vi "MagState.vi"(8 "Error in":errorcluster, 11 "Serial port":refnum<visa-resource-name>="COM28") -> (0 "Error out":errorcluster, 2 "Mag State":bool[](array[boolean]), 3 "Serial port out":refnum<visa-resource-name>)   [LabVIEW 2012]
panel:
  out "State Value":i8[](array[numeric])
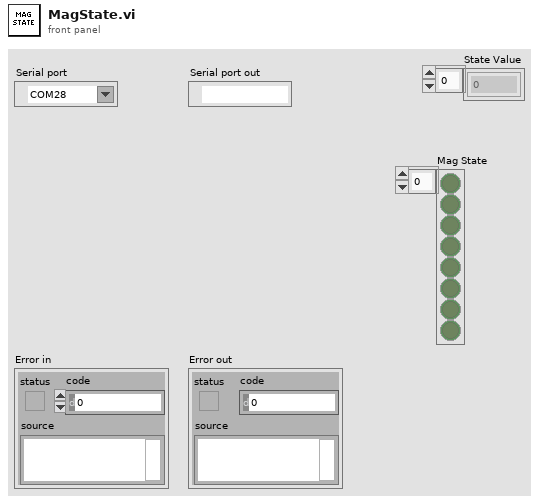
[diagram p1: front panel]
types:
  T1 = enum16{"big-endian, network order", "native, host order", "little-endian"}
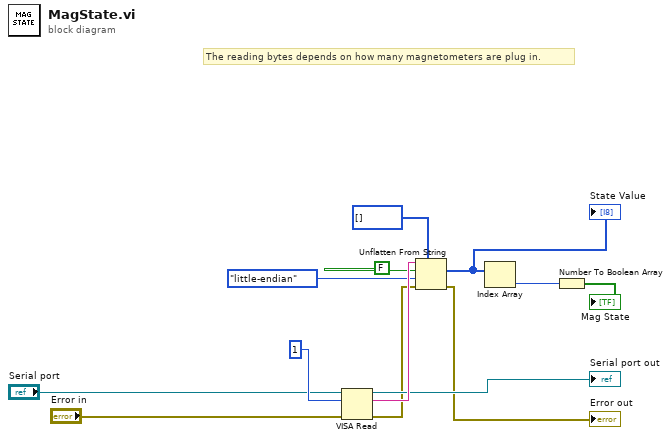
[diagram p0: block diagram]
diagram:
  # "The reading bytes depends on how many magnetometers are plug in."
  n1 = VISA Read(VISA resource name="Serial port", byte count=u32 1, error in (no error)="Error in") -> (VISA resource name out=→"Serial port out":refnum<visa-resource-name>, read buffer=w13:string, error out=w2:errorcluster)  [unwired: 1 out]
  n2 = Unflatten From String(type=i8[] [], binary string=w13, data includes array or string size? (T)=FALSE, byte order (0:big-endian, network order)=T1."little-endian", error in (no error)=w2) -> (value=w7:i8[], error out=→"Error out":errorcluster)  [unwired: 1 out]
  "State Value" <- w7
  n3 = Index Array(array=w7) -> (element=w3:i8)  [unwired: 1 in]
  n4 = Number To Boolean Array(number=w3) -> (Boolean array=→"Mag State":bool[])
